vi "Update Container.vi"(4 "Area Height":u32, 6 "Number of Row":i32, 8 "error in (no error)":errorcluster, 11 "Container Reference":refnum<vi>) -> (0 "error out":errorcluster)   [LabVIEW 2021, in "myRIO Channel List.xctl"]
uses:
  <vilib>/myRIO/Common/Express VI Framework/xctls/myRIO Channel List/myRIO Channel List.xctl
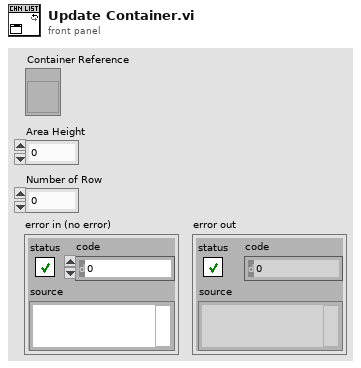
[diagram p1: front panel]
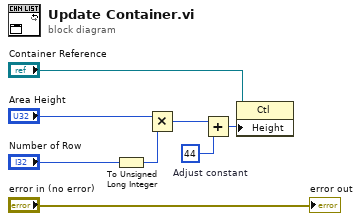
[diagram p0: block diagram]
diagram:
  w3 = u32 44  # Adjust constant
  n1 = To Unsigned Long Integer(number="Number of Row") -> (unsigned 32bit integer=w4:u32)
  n2 = Multiply(x="Area Height", y=w4) -> (x*y=w7:u32)
  n3 = Add(x=w7, y=w3) -> (x+y=w8:u32)
  n4 = property class="Ctl"(reference="Container Reference", "Height"=w8) -> ()  [unwired: 1 in, 2 out]
  "error out" <- "error in (no error)"
